vi "test2.vi"() -> ()   [LabVIEW 2019]
uses:
  <vilib>/Analysis/Matrix/Datatypes/RealMatrix.ctl
  <vilib>/Analysis/Matrix/NI_Matrix.lvlib
panel:
  out "Input A":T1
  out "A":T1
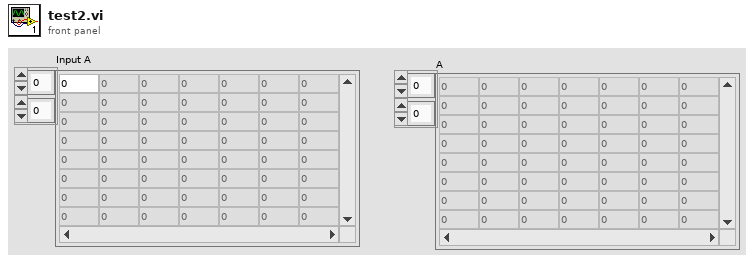
[diagram p1: front panel]
types:
  T1 = typedef "NI_Matrix.lvlib/RealMatrix.ctl" = dbl[][]
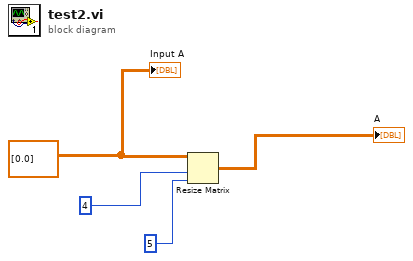
[diagram p0: block diagram]
diagram:
  w4 = T1 [[0.0]] ("input matrix")
  n1 = Resize Matrix(1:5 ("number of columns"), 2:4 ("number of rows"), 4:w4) -> (0:→"A":T1)
  "Input A" <- w4
